vi "U.vi"(11 "Boolean":bool) -> (1 "x = y?":bool)   [LabVIEW 2018]
panel:
  out "number":i32
  out "offset past number":i32
  out "date string":string
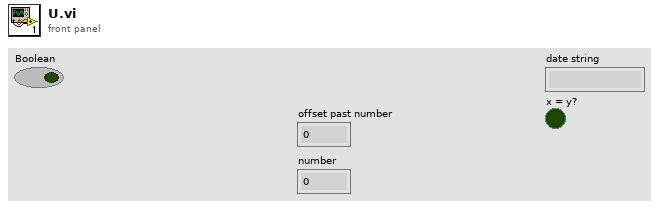
[diagram p1: front panel]
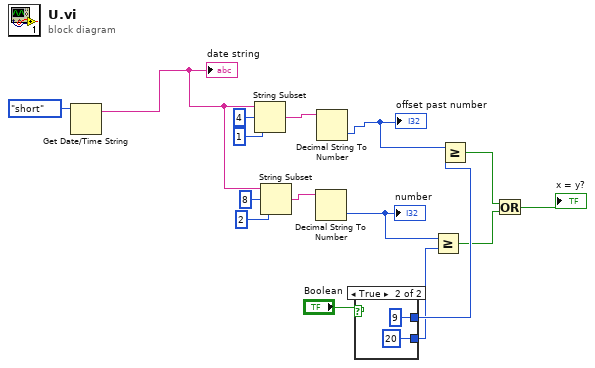
[diagram p0: block diagram]
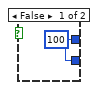
[diagram p2: hidden frame]
diagram:
  n1 = Get Date/Time String(date format (0)=enum16{"short", "long", "abbreviated"}."short") -> (date string=w11:string)  [unwired: 2 in, 1 out]
  "date string" <- w11
  n2 = String Subset(string=w11, offset (0)=4, length (rest)=1 ("length (rest)")) -> (substring=w12:string)
  n3 = String Subset(string=w11, offset (0)=8, length (rest)=2 ("length (rest)")) -> (substring=w8:string)
  n4 = Decimal String To Number(string=w8) -> (number=w2:i32)  [unwired: 2 in, 1 out]
  "number" <- w2
  n5 = Decimal String To Number(string=w12) -> (number=w1:i32)  [unwired: 2 in, 1 out]
  "offset past number" <- w1
  n6 = case shown="True" "Boolean" {
    tunnel: [w17 9] -> w7
    tunnel: [w17 20] -> w6
    frame False {
      w17 = 100
    }
    frame True {
    }
  }
  n7 = Greater Or Equal?(x=w2, y=w6) -> (x >= y?=w4:bool)
  n8 = Greater Or Equal?(x=w1, y=w7) -> (x >= y?=w5:bool)
  n9 = Or(x=w5, y=w4) -> (x .or. y?=→"x = y?":bool)
